vi "Main.vi"() -> ()   [LabVIEW 2014]
uses:
  <vilib>/myRIO/Instrument Drivers/Onboard IO/DIO/typedefs/DIO Reference.ctl
  <vilib>/myRIO/Common/Instrument Driver Framework/Utilities/typedefs/myRIO Generic Hardware Reference.ctl
  <vilib>/myRIO/Common/Instrument Driver Framework/Utilities/typedefs/Hardware Version Enum.ctl
  <vilib>/myRIO/Common/Instrument Driver Framework/Utilities/typedefs/myRIO v1.0 Reference.ctl
  <vilib>/myRIO/Common/Instrument Driver Framework/Utilities/typedefs/Generic FPGA Reference.ctl
  <vilib>/myRIO/Common/Instrument Driver Framework/myRIO v1.0/DIO/typedefs/DIO Channels List.ctl
  <vilib>/myRIO/Common/Instrument Driver Framework/myRIO v1.0/DIO/typedefs/DIO Channels Enum.ctl
  <vilib>/userdefined/High Color/nirio_resource_hc.ctl
  <vilib>/myRIO/Common/Instrument Driver Framework/Utilities/vis/Is FPGA Ref Available.vi
  <vilib>/myRIO/Common/Instrument Driver Framework/myRIO v1.0/DIO/vis/myRIO v1.1 Open DIO.vi
  <vilib>/myRIO/Common/Instrument Driver Framework/myRIO v1.0/PWM/vis/myRIO v1.1 Open PWM.vi
  <vilib>/myRIO/Common/Instrument Driver Framework/Utilities/vis/Validate Channels.vi
  <vilib>/myRIO/Common/Instrument Driver Framework/myRIO v1.0/DIO/vis/myRIO v1.0 Reserve DIO.vi
  <vilib>/myRIO/Common/Instrument Driver Framework/myRIO v1.0/UART/vis/myRIO v1.0 Close UART.vi
  <vilib>/myRIO/Common/Instrument Driver Framework/myRIO v1.0/PWM/vis/myRIO v1.0 Reserve PWM.vi
  <vilib>/myRIO/Common/Instrument Driver Framework/myRIO v1.0/Resource Manager/vis/myRIO v1.0 Reserve Channel List.vi
  <vilib>/myRIO/Common/Instrument Driver Framework/myRIO v1.0/DIO/vis/myRIO v1.0 Build MUX Configuration DIO.vi
  <vilib>/myRIO/Common/Instrument Driver Framework/myRIO v1.0/PWM/vis/myRIO v1.0 Build MUX Configuration PWM.vi
  <vilib>/myRIO/Common/Instrument Driver Framework/myRIO v1.0/Resource Manager/vis/myRIO v1.0 Reserve Channel.vi
  <vilib>/myRIO/Common/Instrument Driver Framework/myRIO v1.0/Resource Manager/vis/myRIO v1.0 Unreserve Channel.vi
  <vilib>/myRIO/Common/Instrument Driver Framework/myRIO v1.0/Resource Manager/vis/myRIO v1.0 Create Configuration List.vi
  <vilib>/myRIO/Common/Instrument Driver Framework/myRIO v1.0/Resource Manager/vis/myRIO v1.0 Build Mutex Name.vi
  <vilib>/Utility/VariantDataType/GetNumericInfo.vi
  <vilib>/Utility/error.llb/Error Cluster From Error Code.vi
  <vilib>/myRIO/Common/Instrument Driver Framework/myRIO v1.0/myRIO v1.1 Open.vi
  <vilib>/myRIO/Common/Instrument Driver Framework/Utilities/vis/IO Manager.vi
  <vilib>/myRIO/Common/Instrument Driver Framework/Utilities/vis/Configuration Manager.vi
  <vilib>/myRIO/Common/Instrument Driver Framework/myRIO v1.0/Resource Manager/vis/myRIO v1.0 Configure IO.vi
  <vilib>/myRIO/Common/Instrument Driver Framework/myRIO v1.0/myRIO v1.0 Close.vi
  <vilib>/myRIO/Common/Instrument Driver Framework/myRIO v1.0/DIO/vis/myRIO v1.0 Write DIO.vi
  <vilib>/myRIO/Common/Instrument Driver Framework/myRIO v1.0/PWM/vis/myRIO v1.0 Write PWM.vi
  <vilib>/myRIO/Common/Instrument Driver Framework/Utilities/vis/FPGA Ref Manager.vi
  <vilib>/myRIO/Common/Instrument Driver Framework/myRIO v1.0/myRIO v1.0 Reset FPGA.vi
  <vilib>/myRIO/Common/Instrument Driver Framework/myRIO v1.0/IRQ/vis/myRIO v1.0 IRQ Info FGV.vi
  <vilib>/myRIO/Common/Instrument Driver Framework/myRIO v1.0/IRQ/vis/myRIO v1.0 Timer IRQ Info FGV.vi
  <vilib>/myRIO/Common/Instrument Driver Framework/myRIO v1.0/IRQ/vis/myRIO v1.0 ISR Agent.vi
  <vilib>/myRIO/Express VI/Onboard Devices/LED/LED Express VI.xnode
  <vilib>/myRIO/Instrument Drivers/Onboard IO/DIO/vis/myRIO DIO Open.xnode
  <vilib>/myRIO/Instrument Drivers/Utilities/Utilities.lvlib
  <vilib>/myRIO/Instrument Drivers/Onboard IO/PWM/PWM.lvlib
  <vilib>/MediaMongrels Ltd/WebSockets/WebSockets/WebSockets.lvlib
  <vilib>/myRIO/Instrument Drivers/Onboard IO/DIO/DIO.lvlib
panel:
  out "Numeric":dbl
  in  "position [%FS]":dbl(slide) scale=-200.0..200.0
  out "Request URI 2":string
  out "HTTP Headers 2":variant
  out "Received Data":string
  in  "Stop":bool
  in  "Send":bool
  in  "Data":string
  in  "position [%FS] 2":dbl(slide) scale=-200.0..200.0
  out "duty cycle [%] 2":dbl
  out "pulse width [ms] 2":dbl=1.5
  out "duty cycle [%]":dbl
  out "pulse width [ms]":dbl=1.5
  out "error out":errorcluster
  in  "Stop Button":bool
  # "Overview: The myRIO Project template acquires acceleration data from the onboard accelerometer and displays the changes of acceleration values in a waveform chart.\nInstructions:\n1. Check the myRIO target IP Address in the project and make sure the target IP Address is correct. \n2. Run the VI."
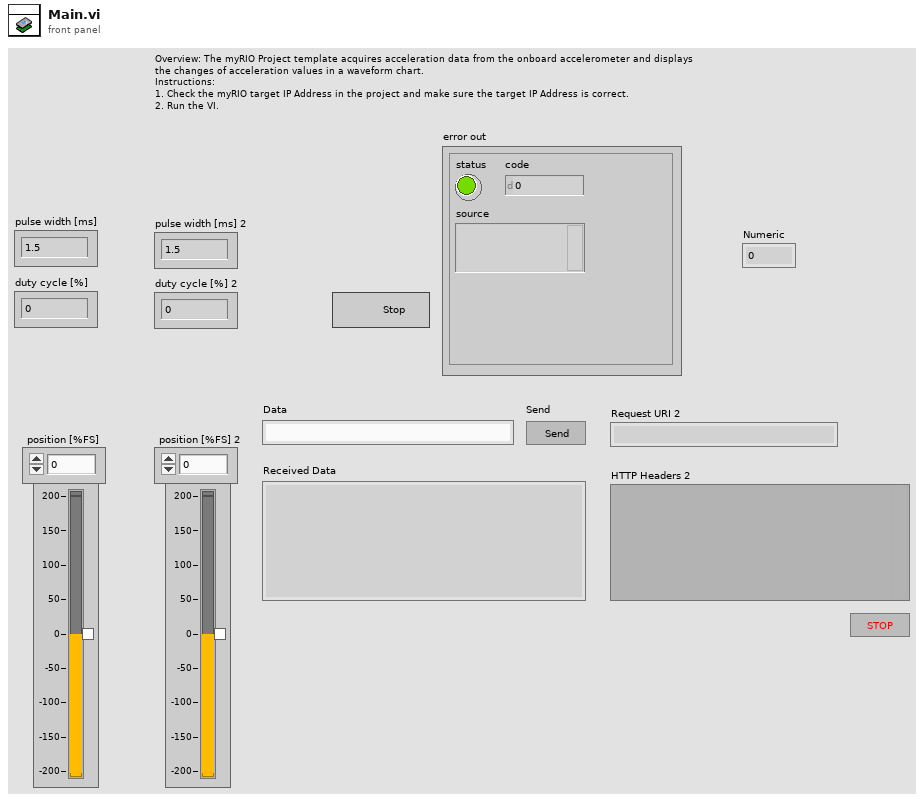
[diagram p1: front panel]
types:
  T1 = typedef "DIO.lvlib/DIO Reference.ctl" = cluster{"myRIO Reference":T2, "DIO Channels List":T6}
  T2 = typedef "myRIO Generic Hardware Reference.ctl" = cluster{"myRIO Model":T3, "myRIO Hardware Reference":T4}
  T3 = typedef "Hardware Version Enum.ctl" = enum16{"Unknown", "myRIO-1900", "myRIO-1950"}
  T4 = typedef "myRIO v1.0 Reference.ctl" = cluster{"Generic FPGA Reference":T5, "Allow multiple opens":bool}
  T5 = typedef "Generic FPGA Reference.ctl" = refnum<k20>
  T6 = typedef "DIO Channels List.ctl" = T7[]
  T7 = typedef "DIO Channels Enum.ctl" = enum16{"Not Connected", "C/DIO0", "C/DIO1", "C/DIO2", "C/DIO3", "C/DIO4", "C/DIO5", "C/DIO6", "C/DIO7", "A/DIO0", "A/DIO1", "A/DIO2", "A/DIO3", "A/DIO4", "A/DIO5", "A/DIO6", "A/DIO7", "A/DIO8", "A/DIO9", "A/DIO10", "A/DIO11", "A/DIO12", "A/DIO13", "A/DIO14", "A/DIO15", "B/DIO0", "B/DIO1", "B/DIO2", "B/DIO3", "B/DIO4", "B/DIO5", "B/DIO6", "B/DIO7", "B/DIO8", "B/DIO9", "B/DIO10", "B/DIO11", "B/DIO12", "B/DIO13", "B/DIO14", "B/DIO15", "LED0", "LED1", "LED2", "LED3", "Button0"}
  T8 = typedef "nirio_resource_hc.ctl" = tag
  T9 = typedef "PWM.lvlib/PWM Reference.ctl" = cluster{"myRIO Reference":T2, "PWM Channels Enum":T10, "PWM Configuration":T11}
  T10 = typedef "PWM Channels Enum.ctl" = enum16{"Not Connected", "C/PWM0", "C/PWM1", "A/PWM0", "A/PWM1", "A/PWM2", "B/PWM0", "B/PWM1", "B/PWM2"}
  T11 = typedef "PWM.lvlib/PWM Configuration.ctl" = cluster{"Frequency":dbl, "Duty Cycle":dbl}
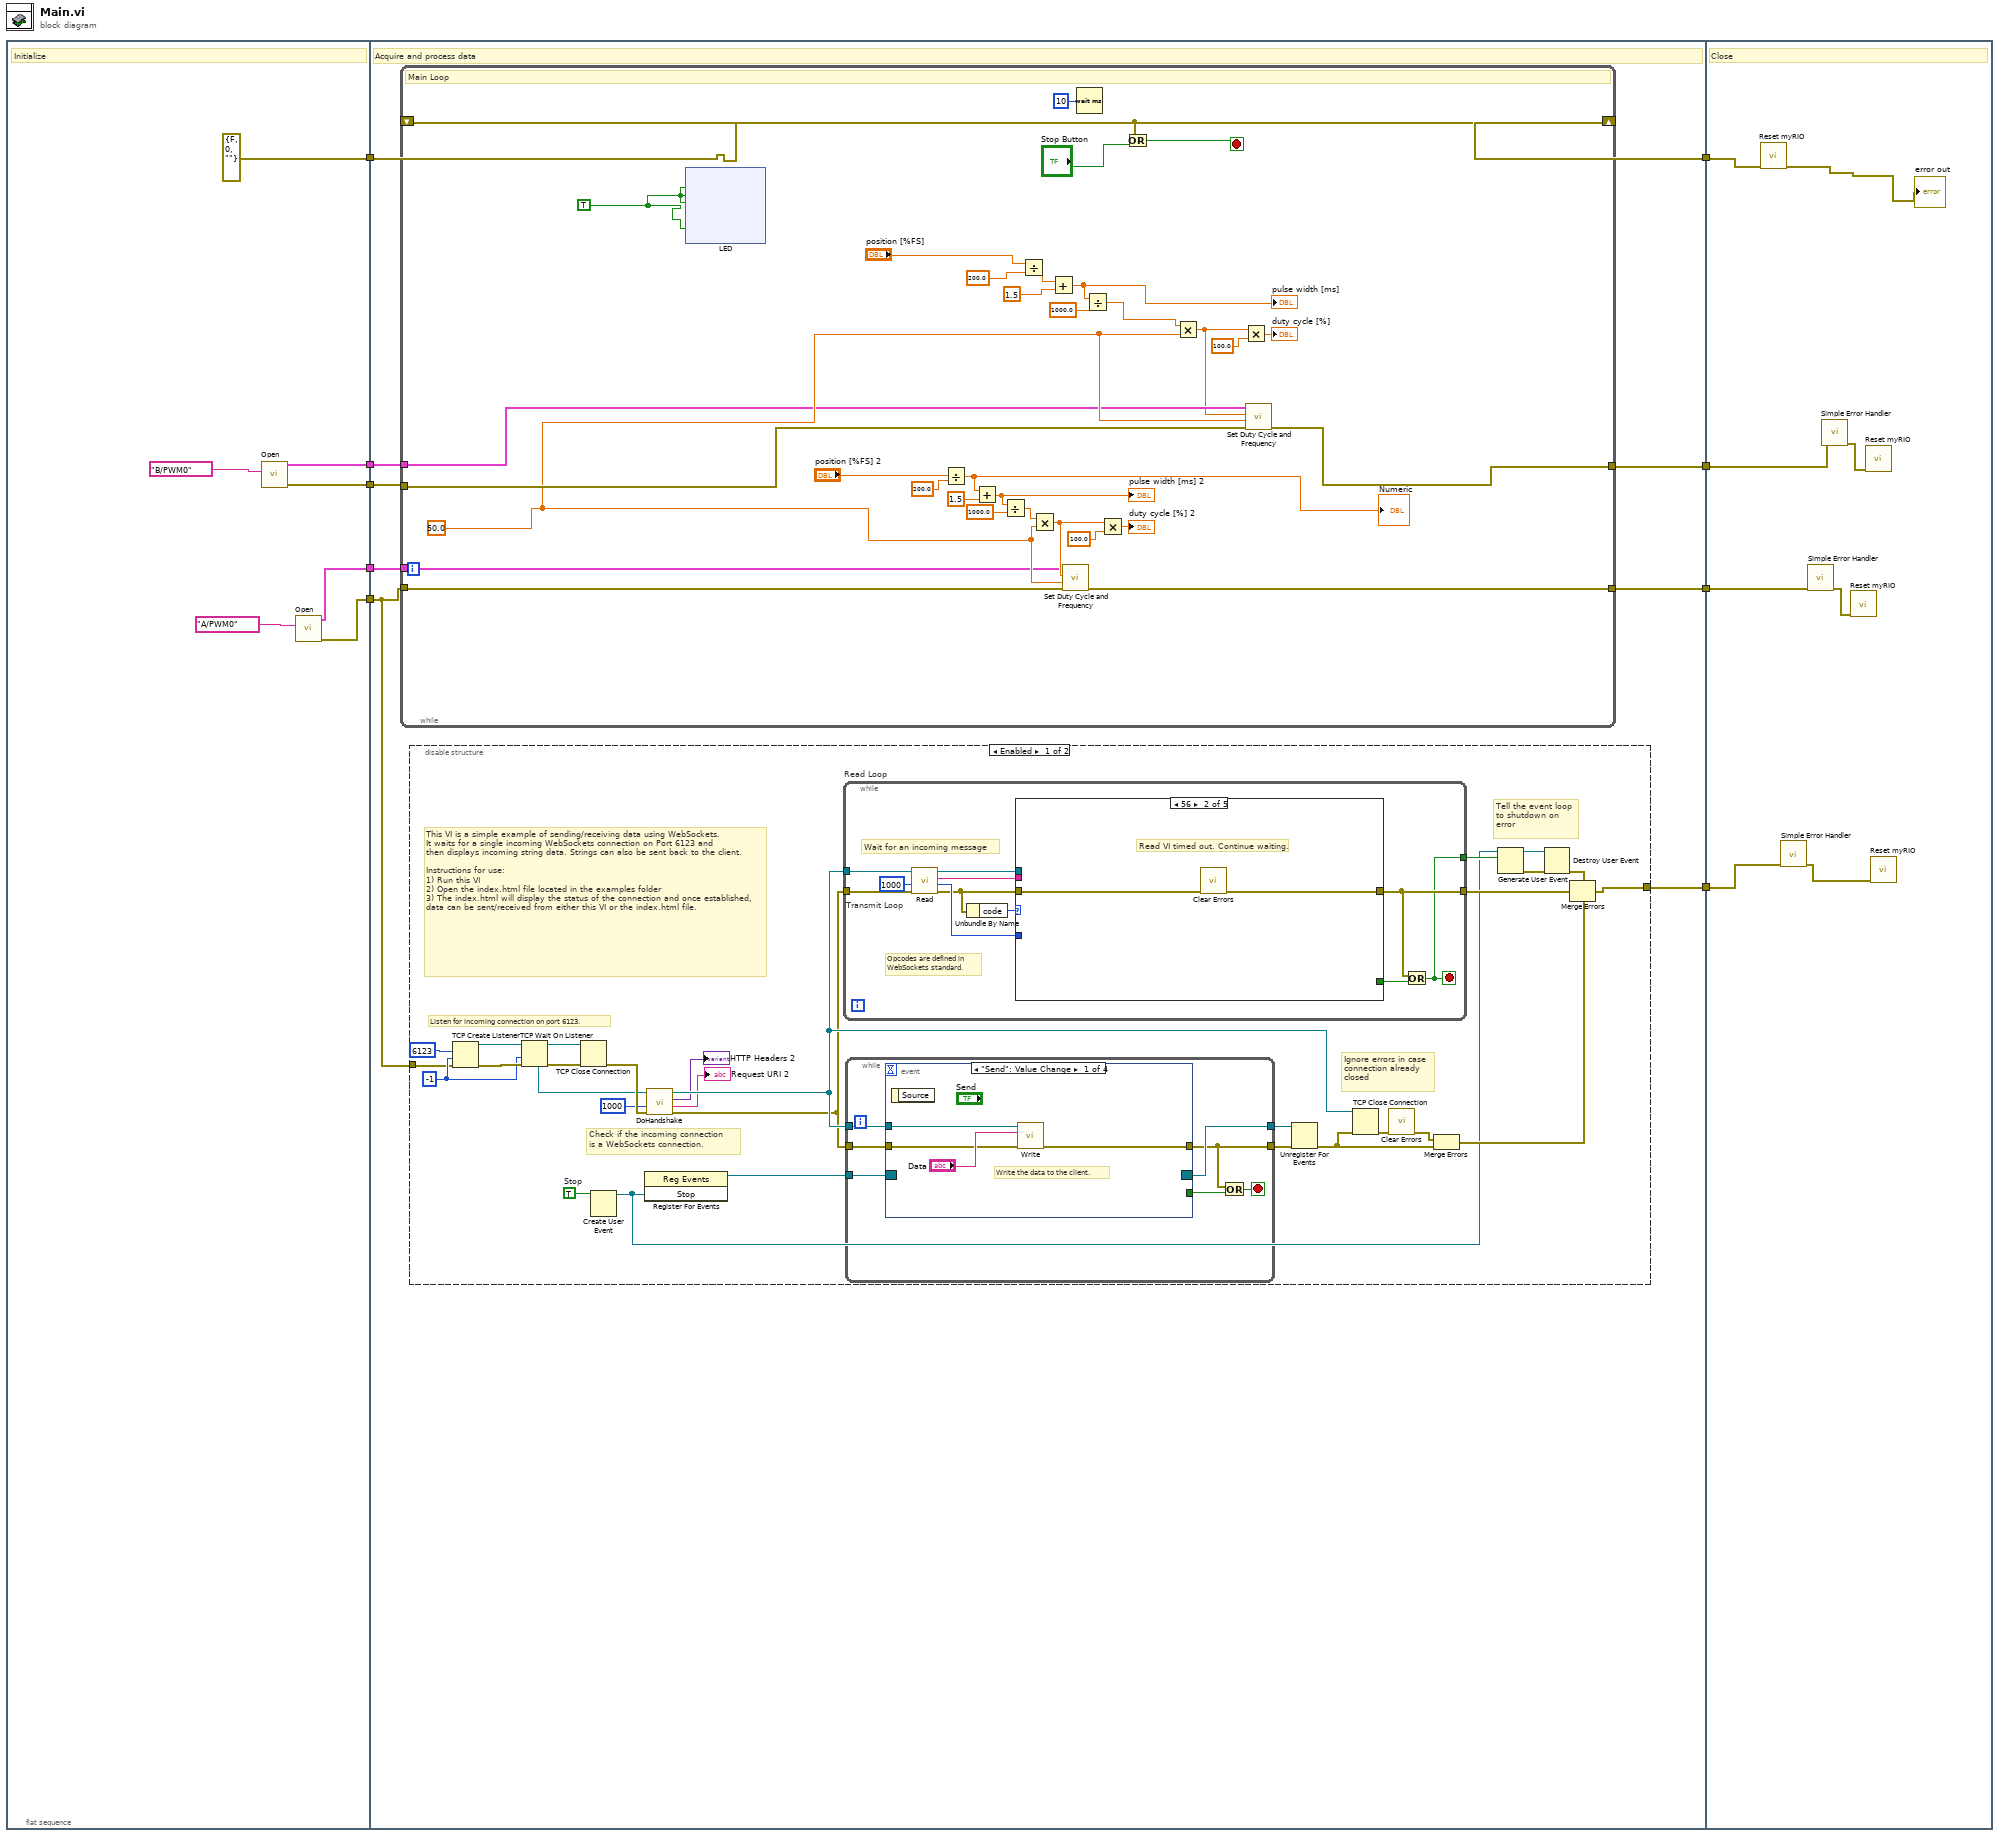
[diagram p0: block diagram]
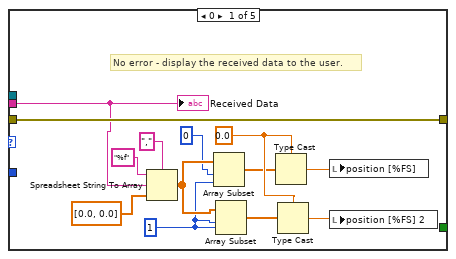
[diagram p2: hidden frame]
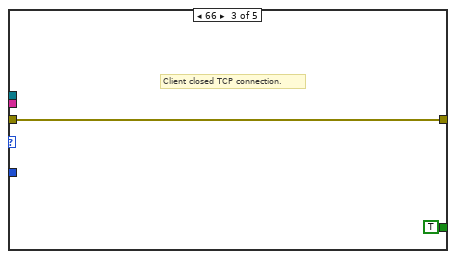
[diagram p3: hidden frame]
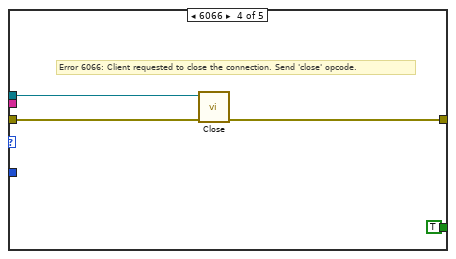
[diagram p4: hidden frame]
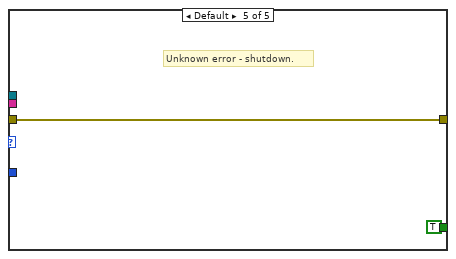
[diagram p5: hidden frame]
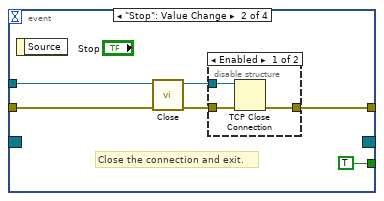
[diagram p6: hidden frame]
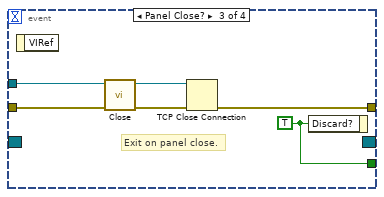
[diagram p8: hidden frame]
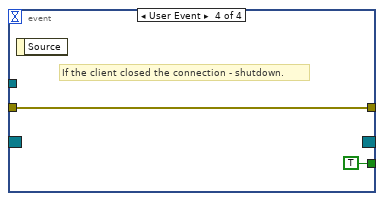
[diagram p9: hidden frame]
diagram:
  n1 = flat-sequence {
    tunnel: [errorcluster {"status"=FALSE, "code"=0, "source"=""} ("error out")] -> w9
    tunnel: [w13] -> w6
    tunnel: [w12] -> w4
    tunnel: [w11] -> w3
    tunnel: [w10] -> w2
    tunnel: w9 -> [w24]
    tunnel: [w25] -> w8
    tunnel: [w23] -> w7
    tunnel: w6 -> [w17]
    tunnel: [w18] -> w5
    tunnel: w4 -> [w20]
    tunnel: w3 -> [w22]
    tunnel: w2 -> [w21]
    tunnel: [w19] -> w1
    tunnel: w8 -> [w194]
    tunnel: w7 -> [w191]
    tunnel: w5 -> [w188]
    tunnel: w1 -> [w189]
    frame #0 {
      # "Initialize"
      n2 = call <vilib>:"Open.vi"("Channel Name"=tag "B/PWM0" ("PWM channel")) -> ("error out"=w10:errorcluster, "PWM Ref Out"=w11:T9)  [unwired: 9 in]
      n3 = call <vilib>:"Open.vi"("Channel Name"=tag "A/PWM0" ("PWM channel 2")) -> ("error out"=w13:errorcluster, "PWM Ref Out"=w12:T9)  [unwired: 9 in]
    }
    frame #1 {
      # "Acquire and process data"
      n4 = while {
        shift-right: [w147] -> w25
        shift-left: w24 -> [w147]
        tunnel: w21 -> [w139]
        tunnel: [w120] -> w23
        tunnel: w17 -> [w130]
        tunnel: w22 -> [w126]
        tunnel: w20 -> [w125]
        tunnel: [w119] -> w19
        stop <- w146 stop-if-true
        w118 = TRUE
        w127 = 50.0
        # "Main Loop"
        n5 = xnode "LED"("LED0"=w118, "LED1"=w118, "LED2"=w118, "LED3"=w118) -> ()  [unwired: 1 in, 1 out]
        n6 = Divide(x="position [%FS] 2", y=200.0) -> (x/y=w117:dbl)
        "Numeric" <- w117
        n7 = Add(x=w117, y=1.5) -> (x+y=w136:dbl)
        "pulse width [ms] 2" <- w136
        n8 = Divide(x=w136, y=1000.0) -> (x/y=w134:dbl)
        n9 = Divide(x="position [%FS]", y=200.0) -> (x/y=w143:dbl)
        n10 = Multiply(x=w134, y=w127) -> (x*y=w131:dbl)
        n11 = Add(x=w143, y=1.5) -> (x+y=w123:dbl)
        "pulse width [ms]" <- w123
        n12 = call <vilib>:"Set Duty Cycle and Frequency.vi"("error in (no error)"=w130, "Frequency [Hz]"=w127, "Duty Cycle"=w131, "PWM Ref In"=w125) -> ("error out"=w119:errorcluster)  [unwired: 5 in, 1 out]
        n13 = Wait (ms)(milliseconds to wait=u32 10) -> ()  [unwired: 1 out]
        n14 = Divide(x=w123, y=1000.0) -> (x/y=w122:dbl)
        n15 = Multiply(x=w131, y=100.0) -> (x*y=→"duty cycle [%] 2":dbl)
        n16 = Or(x=w147, y="Stop Button") -> (x .or. y?=w146:bool)
        n17 = Multiply(x=w122, y=w127) -> (x*y=w124:dbl)
        n18 = Multiply(x=w124, y=100.0) -> (x*y=→"duty cycle [%]":dbl)
        n19 = call <vilib>:"Set Duty Cycle and Frequency.vi"("error in (no error)"=w139, "Frequency [Hz]"=w127, "Duty Cycle"=w124, "PWM Ref In"=w126) -> ("error out"=w120:errorcluster)  [unwired: 5 in, 1 out]
      }
      n20 = disable-structure shown="Enabled" {
        disable-tunnel: [w27 _] -> w18
        disable-tunnel: w17 -> [w26 _]
        frame Enabled {
          w36 = TRUE  # Stop
          w29 = -1 ("timeout ms (25000)")
          # "Ignore errors in case\nconnection already\nclosed"
          # "Tell the event loop to shutdown on error"
          # "This VI is a simple example of sending/receiving data using WebSockets.\nIt waits for a single incoming WebSockets connection on Port 6123 and\nthen displays incoming string data. Strings can also be sent back to the client.\n\nInstructions for use:\n1) Run this VI\n2) Open the index.html file located in the examples folder\n3) The index.html will display the status of the connection and once established, data can be sent/received from either this VI or the index.html file."
          # "Check if the incoming connection\nis a WebSockets connection."
          # "Listen for incoming connection on port 6123."
          n21 = TCP Create Listener(8:w26, 9:w29, 10:u16 6123 ("port")) -> (0:w31:errorcluster, 3:w30:refnum<k5>)  [unwired: 2 in, 1 out]
          n22 = TCP Wait On Listener(8:w31, 9:w29, 11:w30) -> (0:w34:errorcluster, 3:w33:refnum<k5>, 4:w32:refnum<k5>)  [unwired: 1 in, 2 out]
          n23 = TCP Close Connection(connection ID=w33, error in (no error)=w34) -> (error out=w47:errorcluster)  [unwired: 1 in, 1 out]
          n24 = Create User Event(user event datatype=w36) -> (user event=w38:refnum<user-event>)  [unwired: 1 in, 1 out]
          n25 = register-events(w38) -> (reference out=w35:refnum<event-registration>)  [unwired: 2 in, 1 out]
          n26 = call <vilib>:"DoHandshake.vi"("error in (no error)"=w47, "timeout ms (5000)"=1000 ("timeout ms (25000)"), "WebSocket Connection in"=w32) -> ("error out"=w48:errorcluster, "Request URI"=→"Request URI 2":string, "Headers Out"=→"HTTP Headers 2":variant, "WebSocket Connection out"=w50:refnum<k5>)  [unwired: 5 in]
          n27 = while "Read Loop" {
            tunnel: w50 -> [w65]
            tunnel: [w55] -> w39
            tunnel: [w57] -> w49
            tunnel: w48 -> [w58]
            stop <- w55 stop-if-true
            # "Wait for an incoming message"
            # "Opcodes are defined in\nWebSockets standard."
            n28 = call <vilib>:"Read.vi"("error in (no error)"=w58, "timeout ms (5000)"=1000 ("timeout ms (25000)"), "WebSocket Connection in"=w65) -> ("error out"=w59:errorcluster, "Opcode"=w60:u8, "Data"=w62:string, "WebSocket Connection out"=w61:refnum<k5>)  [unwired: 5 in]
            n29 = Unbundle By Name(w59) -> ("code"=w63:i32)
            n30 = case shown="56" w63 {
              tunnel: w62 -> [w75 _ _ _ _]
              tunnel: [_ _ TRUE TRUE TRUE] -> w56
              tunnel: w61 -> [_ _ _ w86 _]
              tunnel: w60 -> [_ _ _ _ _]
              tunnel: w59 -> [w78 w80 w81 w84 w87]
              tunnel: [w78 w79 w81 w83 w87] -> w57
              frame 0 {
                w69 = 1
                w73 = 0.0
                # "No error - display the received data to the user."
                n31 = Spreadsheet String To Array(delimiter (Tab)=",", format string="%f", spreadsheet string=w75, array type (2D Dbl)=dbl[] [0.0, 0.0]) -> (array=w70:dbl[])
                n32 = Array Subset(array=w70, index=0, length=w69) -> (w71:dbl[])
                n33 = Array Subset(array=w70, index=w69, length=w69) -> (w67:dbl[])
                n34 = Type Cast(type=w73, x=w71) -> (*(type *) &x=w72:dbl)
                n35 = Type Cast(type=w73, x=w67) -> (*(type *) &x=w66:dbl)
                n36 = local write "position [%FS]"(w72) -> ()
                n37 = local write "position [%FS] 2"(w66) -> ()
                "Received Data" <- w75
              }
              frame 56 {
                # "Read VI timed out. Continue waiting."
                n38 = call <vilib>:"Clear Errors.vi"("error in (no error)"=w80) -> ("error out"=w79:errorcluster)  [unwired: 5 in, 1 out]
              }
              frame 66 {
                # "Client closed TCP connection."
              }
              frame 6066 {
                # "Error 6066: Client requested to close the connection. Send 'close' opcode."
                n39 = call <vilib>:"Close.vi"("error in (no error)"=w84, "WebSocket Connection in"=w86) -> ("error out"=w83:errorcluster)  [unwired: 8 in, 1 out]
              }
              frame Default {
                # "Unknown error - shutdown."
              }
            }
            n40 = Or(x=w57, y=w56) -> (x .or. y?=w55:bool)
          }
          n41 = while "Transmit Loop" {
            tunnel: w50 -> [w95]
            tunnel: w35 -> [w94]
            tunnel: [w93] -> w37
            tunnel: [w89] -> w46
            tunnel: w48 -> [w92]
            stop <- w90 stop-if-true
            n42 = event shown="[0] \"Send\": Value Change" {
              selector: w94 -> [_ _ _ _]
              dyn-events: [_ _ _ _] -> w93
              timeout: _ -> [_ _ _ _]
              tunnel: w95 -> [w99 w104 w114 _]
              tunnel: [_ TRUE w112 TRUE] -> w91
              tunnel: [w96 w102 w110 w115] -> w89
              tunnel: w92 -> [w97 w100 w109 w115]
              event "Send": Value Change {
                # "Write the data to the client."
                n43 = event-data() -> ()  [unwired: 1 in, 1 out]
                n44 = call <vilib>:"Write.vi"("error in (no error)"=w97, "Data"="Data", "WebSocket Connection in"=w99) -> ("error out"=w96:errorcluster)  [unwired: 7 in, 1 out]
              }
              event "Stop": Value Change {
                # "Close the connection and exit."
                n45 = event-data() -> ()  [unwired: 1 in, 1 out]
                n46 = call <vilib>:"Close.vi"("error in (no error)"=w100, "WebSocket Connection in"=w104) -> ("error out"=w101:errorcluster, "WebSocket Connection in"=w103:refnum<k5>)  [unwired: 8 in]
                n47 = disable-structure shown="Enabled" {
                  disable-tunnel: w103 -> [w108 _]
                  disable-tunnel: [w107 _] -> w102
                  disable-tunnel: w101 -> [w106 _]
                  frame Enabled {
                    n48 = TCP Close Connection(connection ID=w108, error in (no error)=w106) -> (error out=w107:errorcluster)  [unwired: 1 in, 1 out]
                  }
                  frame Disabled {
                  }
                }
              }
              event Panel Close? {
                w112 = TRUE ("Discard?")
                # "Exit on panel close."
                n49 = event-data() -> ()  [unwired: 1 in, 1 out]
                n50 = call <vilib>:"Close.vi"("error in (no error)"=w109, "WebSocket Connection in"=w114) -> ("error out"=w111:errorcluster, "WebSocket Connection in"=w113:refnum<k5>)  [unwired: 8 in]
                n51 = TCP Close Connection(connection ID=w113, error in (no error)=w111) -> (error out=w110:errorcluster)  [unwired: 1 in, 1 out]
                n52 = event-data("Discard?"=w112) -> ()  [unwired: 1 in, 1 out]
              }
              event User Event {
                # "If the client closed the connection - shutdown."
                n53 = event-data() -> ()  [unwired: 1 in, 1 out]
              }
            }
            n54 = Or(x=w89, y=w91) -> (x .or. y?=w90:bool)
          }
          n55 = Unregister For Events(event registration refnum=w37, error in=w46) -> (error out=w52:errorcluster)
          n56 = TCP Close Connection(connection ID=w50, error in (no error)=w52) -> (error out=w51:errorcluster)  [unwired: 1 in, 1 out]
          n57 = call <vilib>:"Clear Errors.vi"("error in (no error)"=w51) -> ("error out"=w54:errorcluster)  [unwired: 5 in, 1 out]
          n58 = Merge Errors(w54, w52) -> (w53:errorcluster)
          n59 = Generate User Event(user event=w38, event data cluster=w39) -> (user event out=w40:refnum<user-event>, error out=w41:errorcluster)  [unwired: 2 in]
          n60 = Destroy User Event(user event=w40, error in=w41) -> (error out=w42:errorcluster)
          n61 = Merge Errors(w42, w49, w53) -> (w27:errorcluster)
        }
        frame Disabled {
        }
      }
    }
    frame #2 {
      # "Close"
      n62 = call <vilib>:"Reset myRIO.vi"("error in (no error)"=w194) -> ("error out"=→"error out":errorcluster)  [unwired: 10 in]
      n63 = call <vilib>:"Simple Error Handler.vi"("error in (no error)"=w188) -> ("error out"=w187:errorcluster)  [unwired: 4 in, 4 out]
      n64 = call <vilib>:"Simple Error Handler.vi"("error in (no error)"=w189) -> ("error out"=w190:errorcluster)  [unwired: 4 in, 4 out]
      n65 = call <vilib>:"Simple Error Handler.vi"("error in (no error)"=w191) -> ("error out"=w192:errorcluster)  [unwired: 4 in, 4 out]
      n66 = call <vilib>:"Reset myRIO.vi"("error in (no error)"=w190) -> ()  [unwired: 10 in, 1 out]
      n67 = call <vilib>:"Reset myRIO.vi"("error in (no error)"=w192) -> ()  [unwired: 10 in, 1 out]
      n68 = call <vilib>:"Reset myRIO.vi"("error in (no error)"=w187) -> ()  [unwired: 10 in, 1 out]
    }
  }
